vi "AssertsGreater.vi"() -> (15 "error out":errorcluster)   [LabVIEW 2016, in "DronaTest.lvlib"]
uses:
  APIs/Assert/AssertControlValue/Greater.vi
  <vilib>/addons/_JKI Toolkits/Caraya/classes/Assert/Assert Not Error.vi
  <vilib>/addons/_JKI Toolkits/Caraya/classes/Assert/Assert Error.vi
  APIs/Assert/AssertControlValue/GreaterOrEqual.vi
  DronaTest.lvlib
  <vilib>/addons/_JKI Toolkits/Caraya/classes/Test/Test.lvclass
  Drona.lvlib
  <vilib>/addons/_JKI Toolkits/Caraya/classes/Assert/Assert.lvclass
  APIs/Assert/AssertControlValue/AssertControlValue.lvlib
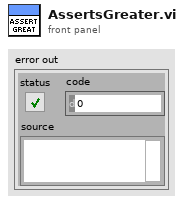
[diagram p1: front panel]
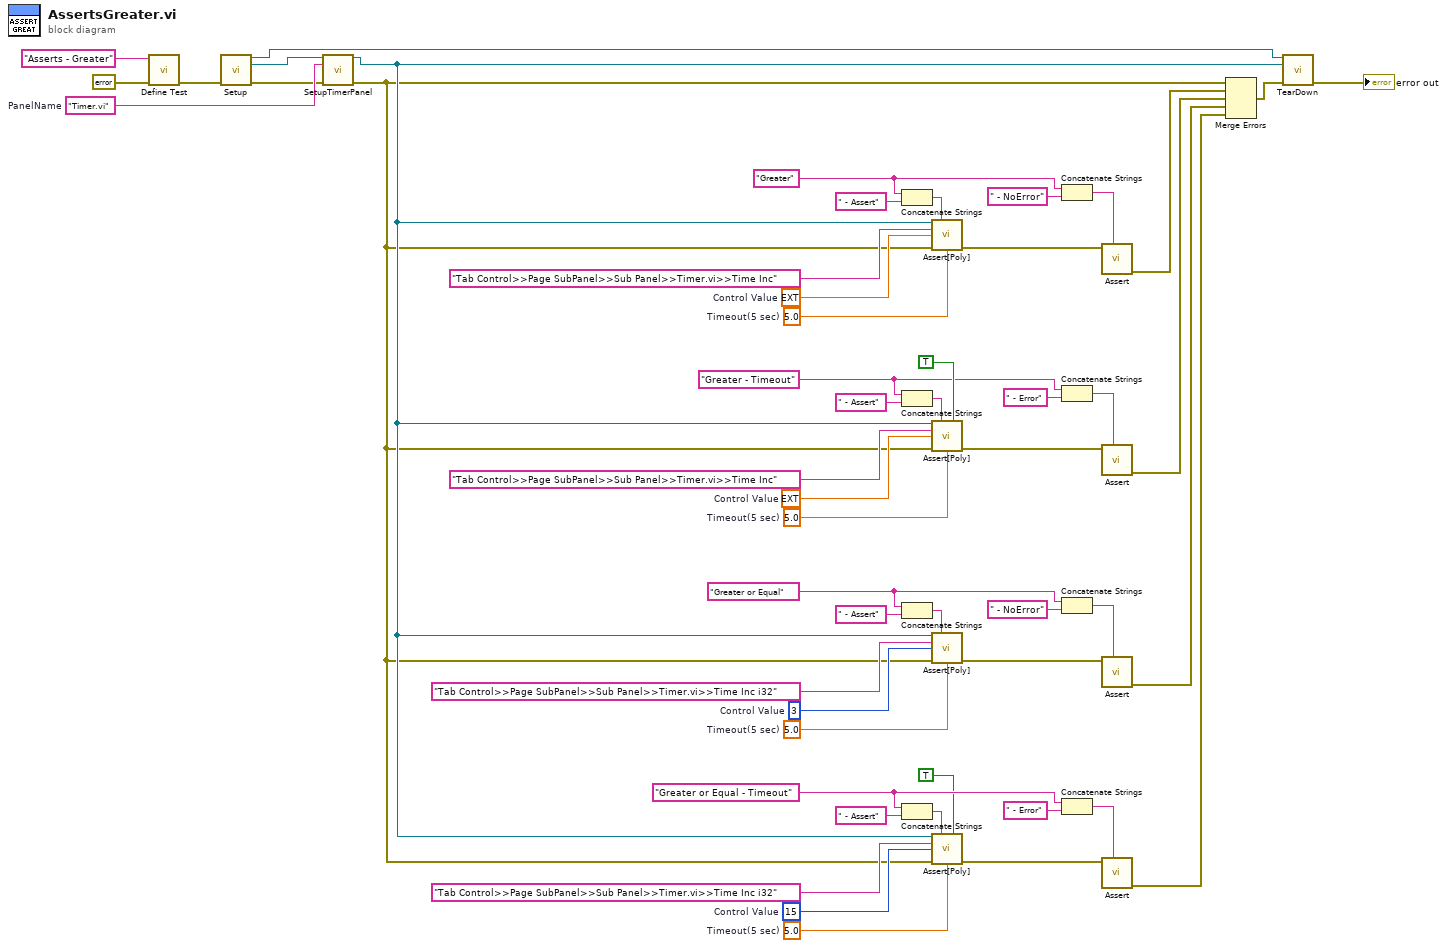
[diagram p0: block diagram]
diagram:
  w9 = "Timer.vi"  # PanelName
  w22 = 5.0  # Timeout(5 sec)
  w23 = 3  # Control Value
  w24 = "Greater or Equal" ("string")
  w21 = 5.0  # Timeout(5 sec)
  w20 = 15  # Control Value
  w19 = "Greater or Equal - Timeout" ("string")
  w39 = 5.0  # Timeout(5 sec)
  w38 = ext 3.0  # Control Value
  w37 = "Greater" ("string")
  w40 = 5.0  # Timeout(5 sec)
  w41 = ext 15.0  # Control Value
  w42 = "Greater - Timeout" ("string")
  n1 = call <vilib>:"Define Test.vi"("error in (no error)"=errorcluster {"status"=FALSE, "code"=0, "source"=""}, "Label (VI Title)"="Asserts - Greater") -> ("error out"=w6:errorcluster)  [unwired: 9 in]
  n2 = call "Setup.vi"("error in (no error)"=w6) -> ("Application Ref"=w5:refnum<vi>, "VI out"=w7:refnum<vi>, "error out"=w8:errorcluster)  [unwired: 12 in]
  n3 = call "SetupTimerPanel.vi"("VI in"=w7, "Panel Name"=w9, "error in (no error)"=w8) -> ("VI out"=w2:refnum<vi>, "error out"=w1:errorcluster)  [unwired: 11 in]
  n4 = Concatenate Strings(w37, " - Assert" ("string")) -> (w35:string)
  n5 = Concatenate Strings(w42, " - Assert" ("string")) -> (w44:string)
  n6 = Concatenate Strings(w24, " - Assert" ("string")) -> (w26:string)
  n7 = Concatenate Strings(w19, " - Assert" ("string")) -> (w17:string)
  n8 = call-poly "Assert[Poly].vi"("VI Reference In"=w2, "Test Label"=w35, "Control Path"="Tab Control>>Page SubPanel>>Sub Panel>>Timer.vi>>Time Inc", "Control Value"=w38, "Error In"=w1, "Timeout(5 sec)"=w39) -> ("Error Out"=w34:errorcluster)  [unwired: 8 in, 1 out]
  n9 = call-poly "Assert[Poly].vi"("VI Reference In"=w2, "Test Label"=w44, "Assert Only? (F)"=TRUE, "Control Path"="Tab Control>>Page SubPanel>>Sub Panel>>Timer.vi>>Time Inc", "Control Value"=w41, "Error In"=w1, "Timeout(5 sec)"=w40) -> ("Error Out"=w45:errorcluster)  [unwired: 7 in, 1 out]
  n10 = call-poly "Assert[Poly].vi"("VI Reference In"=w2, "Test Label"=w26, "Control Path"="Tab Control>>Page SubPanel>>Sub Panel>>Timer.vi>>Time Inc i32", "Control Value"=w23, "Error In"=w1, "Timeout(5 sec)"=w22) -> ("Error Out"=w27:errorcluster)  [unwired: 8 in, 1 out]
  n11 = call-poly "Assert[Poly].vi"("VI Reference In"=w2, "Test Label"=w17, "Assert Only? (F)"=TRUE, "Control Path"="Tab Control>>Page SubPanel>>Sub Panel>>Timer.vi>>Time Inc i32", "Control Value"=w20, "Error In"=w1, "Timeout(5 sec)"=w21) -> ("Error Out"=w16:errorcluster)  [unwired: 7 in, 1 out]
  n12 = Concatenate Strings(w37, " - NoError" ("string")) -> (w36:string)
  n13 = Concatenate Strings(w42, " - Error" ("string")) -> (w43:string)
  n14 = Concatenate Strings(w24, " - NoError" ("string")) -> (w25:string)
  n15 = Concatenate Strings(w19, " - Error" ("string")) -> (w18:string)
  n16 = call-poly <vilib>:"Assert.vi"("Label"=w36, "Not Error?"=w34) -> ("error out"=w51:errorcluster)  [unwired: 9 in]
  n17 = call-poly <vilib>:"Assert.vi"("Label"=w43, "Error?"=w45) -> ("error out"=w50:errorcluster)  [unwired: 9 in]
  n18 = call-poly <vilib>:"Assert.vi"("Label"=w25, "Not Error?"=w27) -> ("error out"=w11:errorcluster)  [unwired: 9 in]
  n19 = call-poly <vilib>:"Assert.vi"("Label"=w18, "Error?"=w16) -> ("error out"=w10:errorcluster)  [unwired: 9 in]
  n20 = Merge Errors(w1, w51, w50, w11, w10) -> (w4:errorcluster)
  n21 = call "TearDown.vi"("Application Ref"=w5, "VI in"=w2, "error in (no error)"=w4) -> ("error out"=→"error out":errorcluster)  [unwired: 12 in]
